vi "Message_dialog.vi"(8 "error in (no error)":errorcluster, 10 "set delay":dbl=5.0, 11 "String":string) -> (0 "error out":errorcluster)   [LabVIEW 2020]
panel:
  out "concatenated string":string
  in  "OK":bool
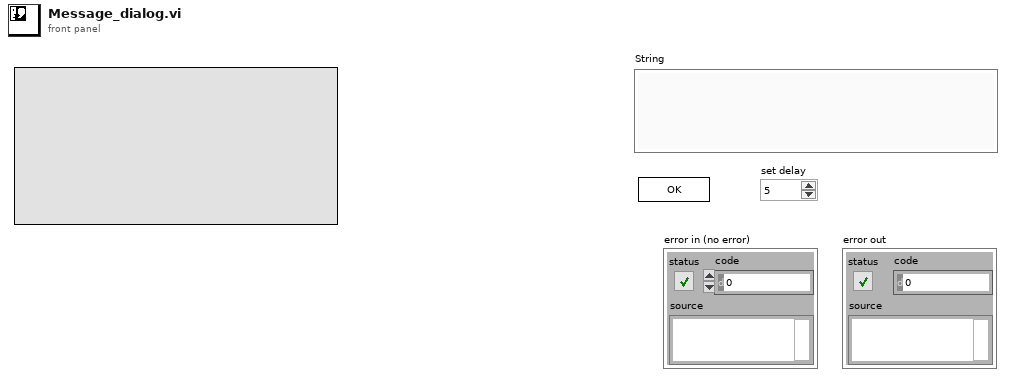
[diagram p1: front panel]
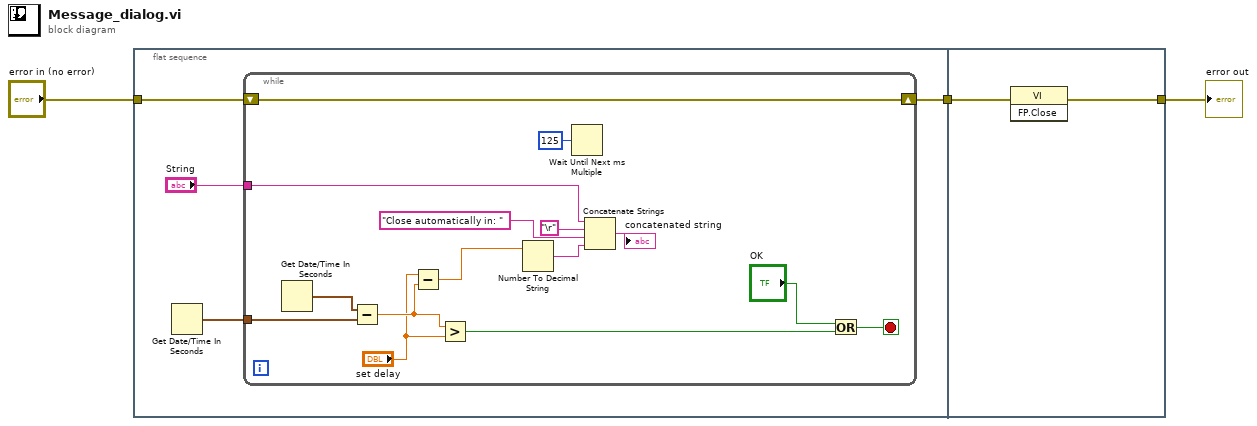
[diagram p0: block diagram]
diagram:
  n1 = flat-sequence {
    tunnel: [w5] -> w3
    tunnel: "error in (no error)" -> [w4]
    tunnel: w3 -> [w24]
    tunnel: [w23] -> w1
    frame #0 {
      n2 = Get Date/Time In Seconds() -> (seconds since 1Jan1904=w7:timestamp)
      n3 = while {
        tunnel: w7 -> [w18]
        tunnel: "String" -> [w10]
        shift-right: [w9] -> w5
        shift-left: w4 -> [w9]
        stop <- w21 stop-if-true
        n4 = Get Date/Time In Seconds() -> (seconds since 1Jan1904=w19:timestamp)
        n5 = Subtract(x=w19, y=w18) -> (x-y=w13:dbl)
        n6 = Subtract(x="set delay", y=w13) -> (x-y=w12:dbl)
        n7 = Greater?(x=w13, y="set delay") -> (0:w17:bool)
        n8 = Number To Decimal String(number=w12) -> (decimal integer string=w15:string)  [unwired: 1 in]
        n9 = Wait Until Next ms Multiple(millisecond multiple=u32 125) -> ()  [unwired: 1 out]
        n10 = Concatenate Strings(w10, "\r", "Close automatically in: ", w15) -> (→"concatenated string":string)
        n11 = Or(x="OK", y=w17) -> (x .or. y?=w21:bool)
      }
    }
    frame #1 {
      n12 = invoke class="VI" method="FP.Close"(error in=w24) -> (error out=w23:errorcluster)  [unwired: 2 in, 2 out]
    }
  }
  "error out" <- w1
